vi "SpeedTest.vi"() -> ()   [LabVIEW 2012]
uses:
  <vilib>/MakerHub/KinectOne/KinectOne.lvlib
  <vilib>/MakerHub/KinectOne/Private/kinectRead [DepthFrame].vi
  Support VIs/ComputeRectAverage.vi
  <vilib>/vision/Image Controls.llb/IMAQ Image.ctl
panel:
  out "Image Out":T1
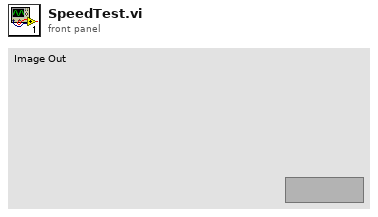
[diagram p1: front panel]
types:
  T1 = typedef "IMAQ Image.ctl" = refnum<image>
  T2 = typedef "KinectOne.lvlib/KinectSensor References.ctl" = cluster{"KinectSensor":refnum<k24>, "MultiSourceFrameReader":refnum<k24>, "BodyFrameDataInterface":refnum<k24>}
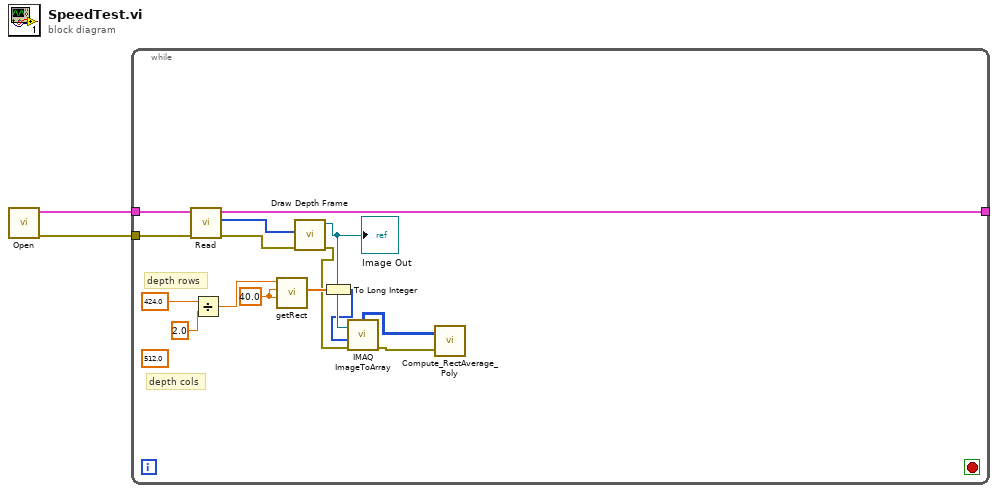
[diagram p0: block diagram]
diagram:
  n1 = call <vilib>:"Open.vi"() -> ("Error Out"=w1:errorcluster, "KinectSensor References out"=w2:T2)  [unwired: 10 in]
  n2 = while {
    tunnel: w2 -> [w17]
    tunnel: w1 -> [w16]
    tunnel: [w15] -> _
    stop <- _ stop-if-true
    w8 = 40.0 ("X")
    (unwired) 512.0
    # "depth rows"
    # "depth cols"
    n3 = call-poly <vilib>:"Read.vi"("Error In"=w16, "KinectSensor References in"=w17) -> ("Error Out"=w13:errorcluster, "frameData"=w14:u16[], "KinectSensor References out"=w15:T2)  [unwired: 7 in]
    n4 = Divide(x=424.0, y=2.0) -> (x/y=w9:dbl)
    n5 = call "getRect.vi"("Y"=w8, "X"=w8, "Offset"=w9) -> ("rect array"=w7:dbl[])  [unwired: 8 in]
    n6 = call <vilib>:"Draw Depth Frame.vi"("Error In"=w13, "U16 Array"=w14) -> ("Error Out"=w6:errorcluster, "Image Out"=w12:T1)  [unwired: 8 in]
    "Image Out" <- w12
    n7 = To Long Integer(number=w7) -> (32bit integer=w4:i32[])
    n8 = call "IMAQ ImageToArray"("error in (no error)"=w6, "Optional Rectangle"=w4, "Image"=w12) -> ("error out"=w5:errorcluster, "Image Pixels (U8)"=w3:u8[][])  [unwired: 1 in, 3 out]
    n9 = call-poly "Compute_RectAverage_Poly.vi"("Error In"=w5, "Image Pixels (U32)"=w3) -> ()  [unwired: 1 in, 4 out]
  }
